vi "Set Exclusions.vi"(4 "Exclude dependent shared libraries":bool, 6 "Exclude dependent packed libraries":bool, 8 "error in (no error)":errorcluster, 9 "Disconnect inline subVIs (F)":bool, 10 "Exclusions":T1={"Disconnect type definitions"=FALSE, "Remove unused polymorphic VI instances"=TRUE, "Remove unused members of project libraries"=TRUE, "Modify project library file after removing unused members"=TRUE}, 11 "PPL in":refnum<class "NI_AB_API_PPL.lvclass">) -> (0 "error out":errorcluster, 3 "PPL out":refnum<class "NI_AB_API_PPL.lvclass">)   [LabVIEW 2020, in "NI_AB_API_PPL.lvclass"]
uses:
  <vilib>/AppBuilder/AB_API/PPL/NI_AB_API_PPL.lvclass
  <vilib>/AppBuilder/AB_API/common/AB_API Primary Exclusions.ctl
  <vilib>/AppBuilder/AB_API/Targetfile/NI_AB_API_Targetfile.lvclass
panel:
  # "^ unsupported for packed project libraries"
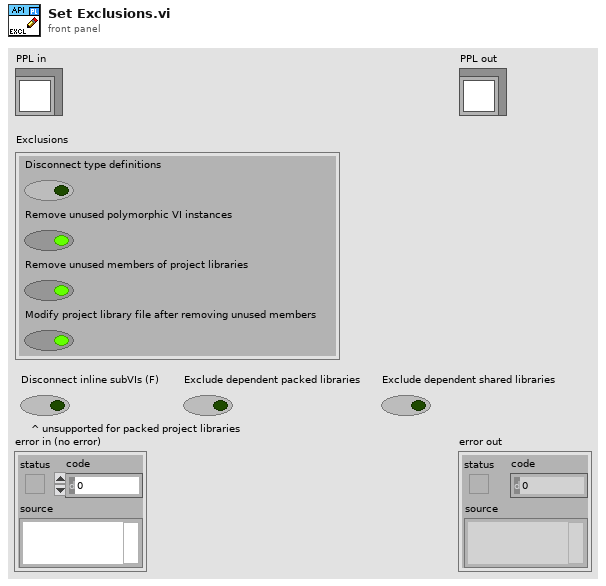
[diagram p1: front panel]
types:
  T1 = typedef "AB_API Primary Exclusions.ctl" = cluster{"Disconnect type definitions":bool, "Remove unused polymorphic VI instances":bool, "Remove unused members of project libraries":bool, "Modify project library file after removing unused members":bool}
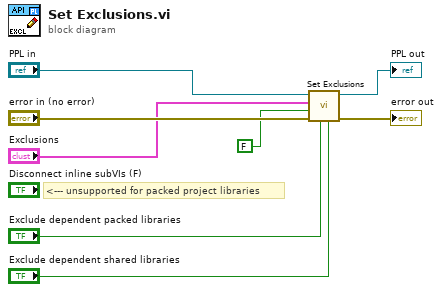
[diagram p0: block diagram]
diagram:
  # "<--- unsupported for packed project libraries"
  n1 = call-parent "Set Exclusions.vi"("Exclude dependent shared libraries"="Exclude dependent shared libraries", "Exclude dependent packed libraries"="Exclude dependent packed libraries", "error in (no error)"="error in (no error)", "Disconnect inline subVIs"=FALSE, "Exclusions"="Exclusions", "Build in"="PPL in") -> ("error out"=→"error out":errorcluster, "Build out"=→"PPL out":refnum<class "NI_AB_API_PPL.lvclass">)  [unwired: 4 in]
